vi "Get Modules Disabled Items.vi"() -> (3 "DisabledItems[]":i32[](array[numeric]))   [LabVIEW 2019, in "Scan Engine Custom Device.lvlib"]
uses:
  Scan Engine Custom Device.lvlib
  Modules.lvlibp/RSI Module/Module Models.ctl
  Modules.lvlibp/RSI Module/Slot Settings.ctl
  Modules.lvlibp/RSI Module/RSI Module.lvclass
  Modules.lvlibp
panel:
  in  "Module":T1
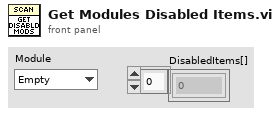
[diagram p1: front panel]
types:
  T1 = typedef "Modules.lvlibp/RSI Module.lvclass/Module Models.ctl" = enum16{"Empty", "NI 9201", "NI 9203", "NI 9205", "NI 9206", "NI 9207", "NI 9208", "NI 9209", "NI 9210", "NI 9211", "NI 9212", "NI 9213", "NI 9214", "NI 9215", "NI 9216", "NI 9217", "NI 9219", "NI 9220", "NI 9221", "NI 9222", "NI 9223", "NI 9224", "NI 9225", "NI 9226", "NI 9227", "NI 9228", "NI 9229", "NI 9233", "NI 9234", "NI 9235", "NI 9236", "NI 9237", "NI 9239", "NI 9242", "NI 9244", "NI 9253", "NI 9263", "NI 9264", "NI 9265", "NI 9266", "NI 9269", "NI 9344", "NI 9350", "NI 9375", "NI 9401", "NI 9402", "NI 9403", "NI 9411", "NI 9421", "NI 9422", "NI 9423", "NI 9425", "NI 9426", "NI 9435", "NI 9436", "NI 9437", "NI 9472", "NI 9474", "NI 9475", "NI 9476", "NI 9477", "NI 9478", "NI 9481", "NI 9482", "NI 9485"}
  T2 = typedef "Modules.lvlibp/RSI Module.lvclass/Slot Settings.ctl" = cluster{"Slot":u32, "EtherCAT?":bool}
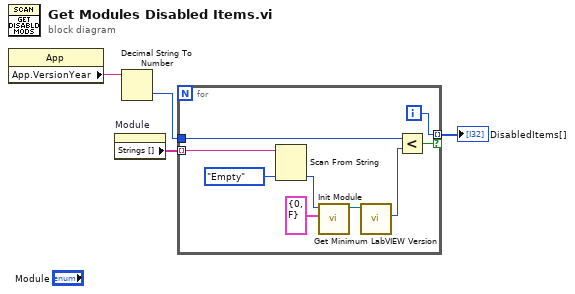
[diagram p0: block diagram]
diagram:
  n1 = property class="App"() -> ("App.VersionYear"=w1:string)  [unwired: 2 in, 2 out]
  n2 = property on="Module" class="Enum (strict)"() -> ("Strings []"=w4:string[])  [unwired: 2 in, 2 out]
  n3 = Decimal String To Number(string=w1) -> (number=w2:i32)  [unwired: 2 in, 1 out]
  n4 = for {
    tunnel: w2 -> [w11]
    tunnel: [w6] -> w3 mode=indexing if=w10
    tunnel: w4 -> [w8] mode=indexing
    i -> [w6]
    n5 = Scan From String(input string=w8, default 1=Module_Models."Empty" ("Model")) -> (output 1=w5:T1)  [unwired: 3 in, 3 out]
    n6 = call "Init Module.vi"("Slot Settings"=T2 {"Slot"=0, "EtherCAT?"=FALSE}, "Module Model"=w5) -> ("RSI Module out"=w12:refnum<class "RSI Module.lvclass">)  [unwired: 8 in, 1 out]
    n7 = call-dynamic "Get Minimum LabVIEW Version.vi"("RSI Module in"=w12) -> ("Minimum LabVIEW Version"=w9:i32)  [unwired: 8 in, 2 out]
    n8 = Less?(x=w11, y=w9) -> (x < y?=w10:bool)
  }
  "DisabledItems[]" <- w3
